vi "Query_Vizier.vi"(6 "Folder":path, 7 "wget":path, 8 "Width":dbl, 9 "Height":dbl, 10 "DEC":dbl, 11 "RA":dbl) -> (1 "error?":bool, 3 "Path2Image":path)   [LabVIEW 2019]
panel:
  out "standard output":string
  out "Final Name":string
  out "CMD Error":errorcluster
  out "standard error":string
  out "rm2 Error":errorcluster
  out "rm error":errorcluster
  out "Img Coords":cluster{"RA":dbl, "DEC":dbl}[](array[cluster]) {"DEC" format="%.2g"; "RA" format="%.2g"}
  out "complete command":string
  out "identifier":string
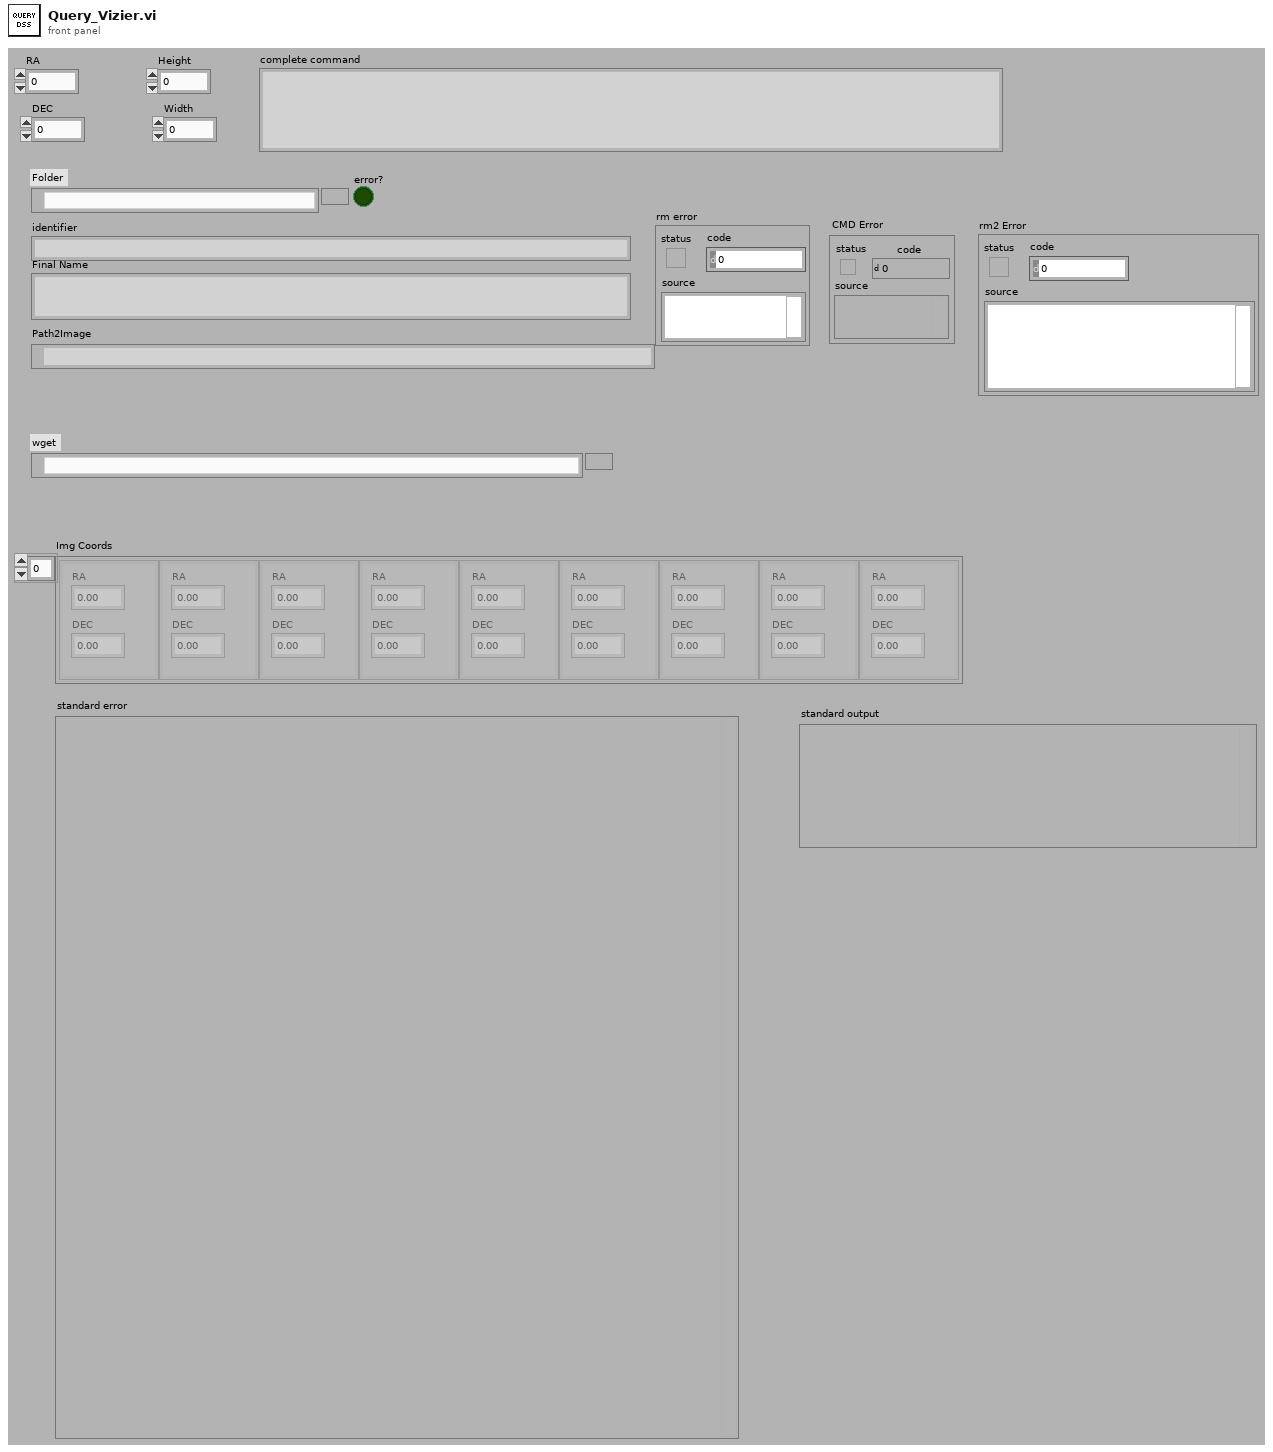
[diagram p1: front panel]
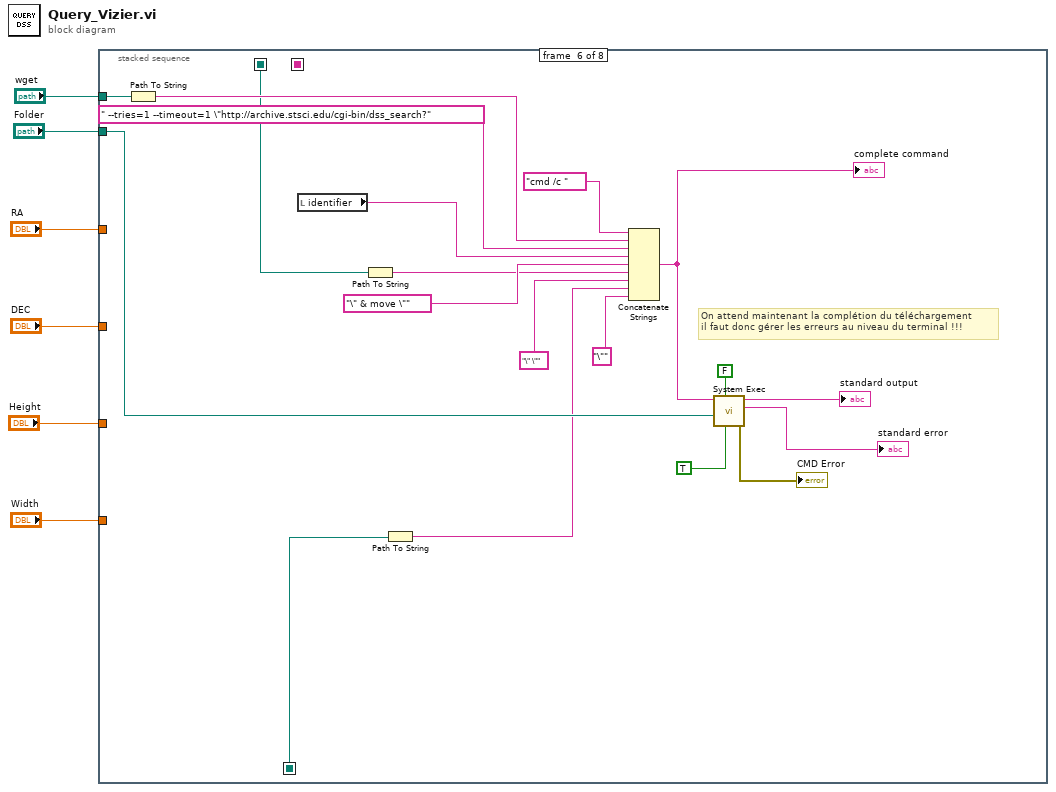
[diagram p0: block diagram]
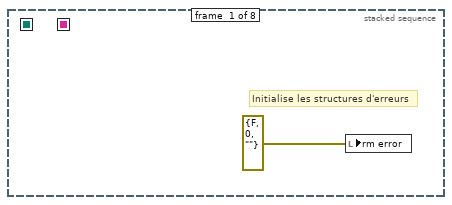
[diagram p2: hidden frame]
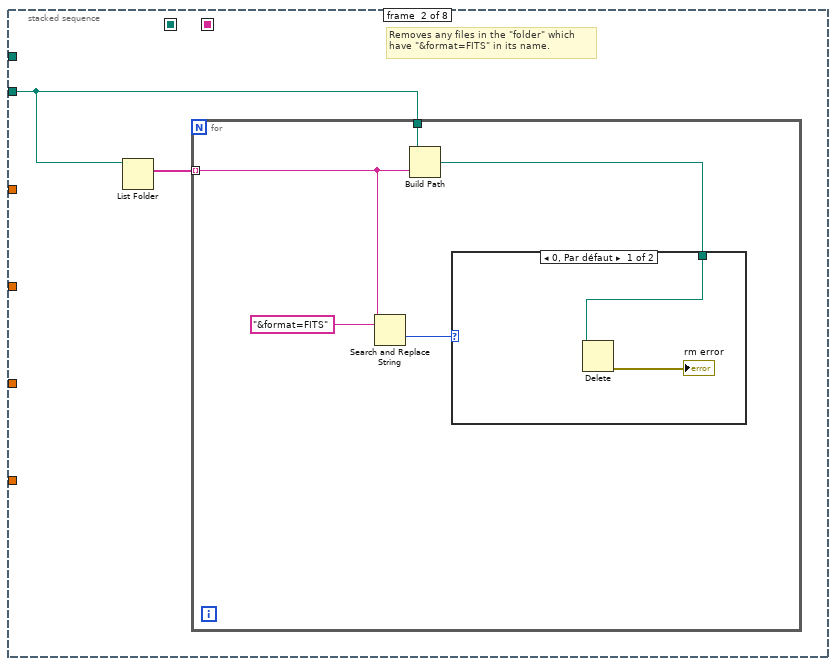
[diagram p3: hidden frame]
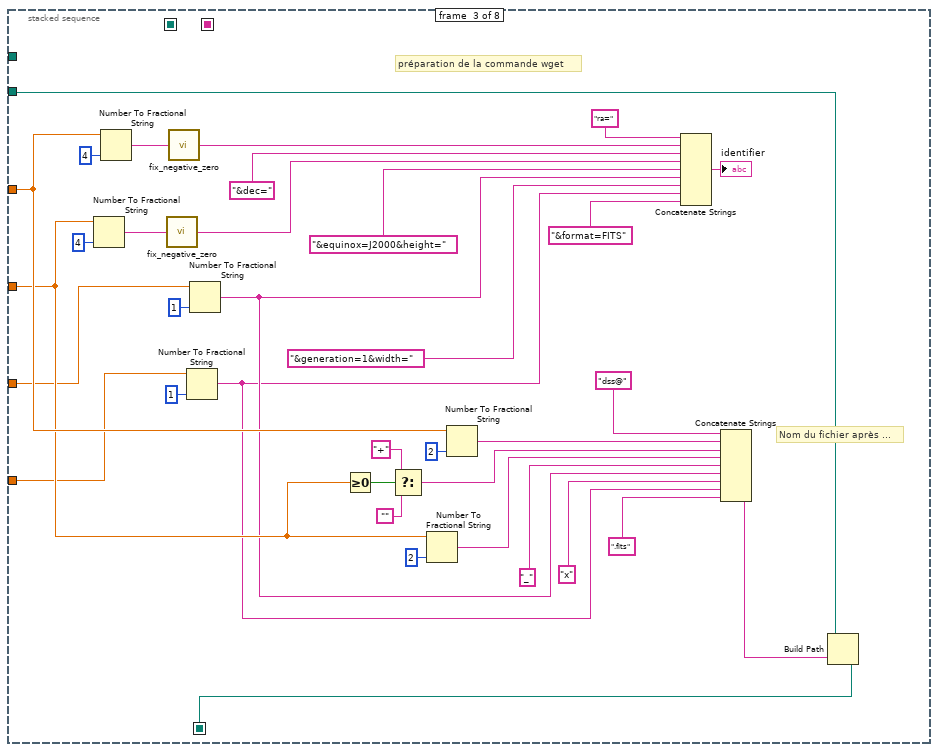
[diagram p5: hidden frame]
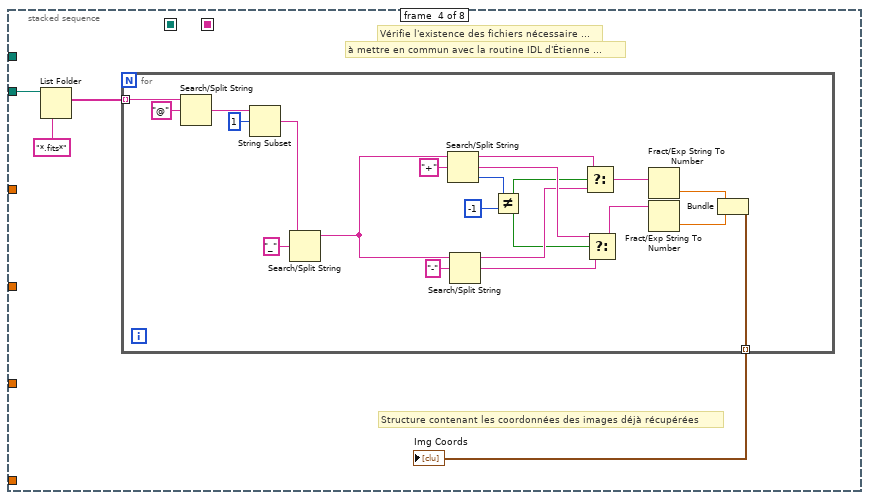
[diagram p6: hidden frame]
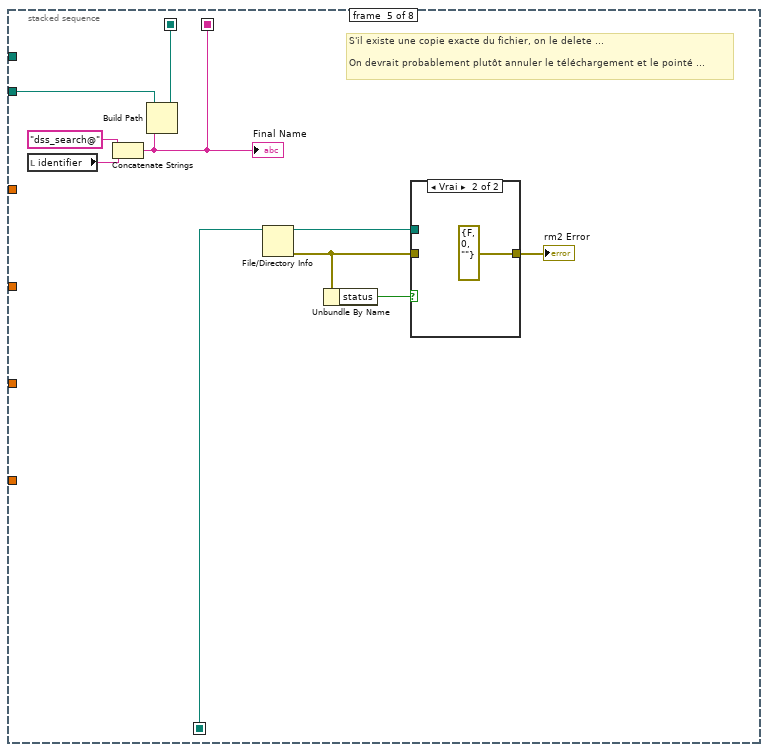
[diagram p7: hidden frame]
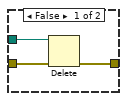
[diagram p8: hidden frame]
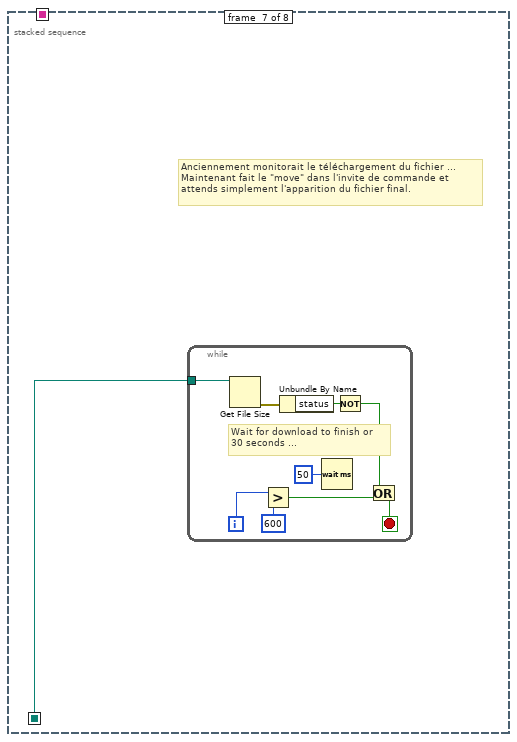
[diagram p9: hidden frame]
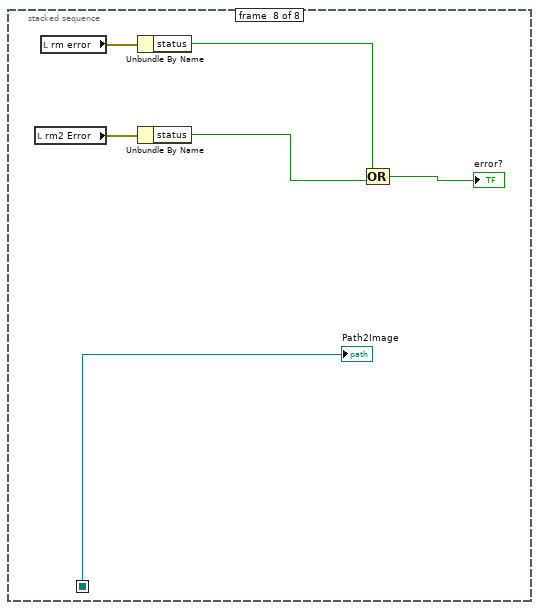
[diagram p10: hidden frame]
diagram:
  n1 = stacked-sequence {
    seq-local: [_ _ w20 _ _ _ _ _] -> [_ _ _ _ w77 w98 w110 w120]
    seq-local: [_ _ _ _ w82 _ _ _] -> [_ _ _ _ _ w97 _ _]
    seq-local: [_ _ _ _ w78 _ _ _] -> [_ _ _ _ _ _ _ _]
    tunnel: "Folder" -> [_ w8 w21 w55 w84 w109 _ _]
    tunnel: "RA" -> [_ _ w31 _ _ _ _ _]
    tunnel: "DEC" -> [_ _ w30 _ _ _ _ _]
    tunnel: "Height" -> [_ _ w29 _ _ _ _ _]
    tunnel: "Width" -> [_ _ w28 _ _ _ _ _]
    tunnel: "wget" -> [_ _ _ _ _ w104 _ _]
    frame #0 {
      # "Initialise les structures d'erreurs"
      n2 = local write "rm error"(errorcluster {"status"=FALSE, "code"=0, "source"=""} ("error out")) -> ()
    }
    frame #1 {
      # "Removes any files in the \"folder\" which\nhave \"&format=FITS\" in its name."
      n3 = List Folder(path=w8) -> (filenames=w9:string[])  [unwired: 3 in, 3 out]
      n4 = for {
        tunnel: w9 -> [w12] mode=indexing
        tunnel: w8 -> [w11]
        n5 = Search and Replace String(input string=w12, search string="&format=FITS") -> (offset past replacement=w13:i32)  [unwired: 6 in, 3 out]
        n6 = Build Path(base path=w11, name or relative path=w12) -> (appended path=w10:path)
        n7 = case shown="0, Par défaut" w13 {
          tunnel: w10 -> [w16 _]
          frame 0, Default {
            n8 = Delete(path (use dialog)=w16) -> (error out=→"rm error":errorcluster)  [unwired: 4 in, 2 out]
          }
          frame -1 {
          }
        }
      }
    }
    frame #2 {
      # "préparation de la commande wget"
      # "Nom du fichier après ..."
      n9 = Number To Fractional String(number=w30, precision (6)=i16 4) -> (F-format string=w33:string)  [unwired: 2 in]
      n10 = Number To Fractional String(number=w31, precision (6)=i16 4) -> (F-format string=w41:string)  [unwired: 2 in]
      n11 = call "fix_negative_zero.vi"("String IN"=w33) -> ("String OUT"=w17:string)
      n12 = call "fix_negative_zero.vi"("String IN"=w41) -> ("String OUT"=w18:string)
      n13 = Number To Fractional String(number=w28, precision (6)=i16 1) -> (F-format string=w23:string)  [unwired: 2 in]
      n14 = Number To Fractional String(number=w29, precision (6)=i16 1) -> (F-format string=w26:string)  [unwired: 2 in]
      n15 = Greater Or Equal To 0?(x=w30) -> (x >= 0?=w47:bool)
      n16 = Select(t="+" ("string"), s=w47, f="" ("string")) -> (s? t:f=w50:string)
      n17 = Number To Fractional String(number=w30, precision (6)=i16 2) -> (F-format string=w46:string)  [unwired: 2 in]
      n18 = Number To Fractional String(number=w31, precision (6)=i16 2) -> (F-format string=w45:string)  [unwired: 2 in]
      n19 = Concatenate Strings("ra=" ("string"), w18, "&dec=" ("string"), w17, "&equinox=J2000&height=" ("string"), w26, "&generation=1&width=" ("string"), w23, "&format=FITS" ("string")) -> (→"identifier":string)
      n20 = Concatenate Strings("dss@" ("string"), w45, w50, w46, "_" ("string"), w26, "x" ("string"), w23, ".fits" ("string")) -> (w22:string)
      n21 = Build Path(base path=w21, name or relative path=w22) -> (appended path=w20:path)
    }
    frame #3 {
      # "Structure contenant les coordonnées des images déjà récupérées"
      # "à mettre en commun avec la routine IDL d'Étienne ..."
      # "Vérifie l'existence des fichiers nécessaire ..."
      n22 = List Folder(path=w55, pattern="*.fits*") -> (filenames=w54:string[])  [unwired: 2 in, 3 out]
      n23 = for {
        tunnel: w54 -> [w76] mode=indexing
        tunnel: [w56] -> w52 mode=indexing
        n24 = Search/Split String(string=w76, search string/char (-)="@") -> (match + rest of string=w73:string)  [unwired: 1 in, 2 out]
        n25 = String Subset(string=w73, offset (0)=1) -> (substring=w71:string)  [unwired: 1 in]
        n26 = Search/Split String(string=w71, search string/char (-)="_") -> (substring before match=w66:string)  [unwired: 1 in, 2 out]
        n27 = Search/Split String(string=w66, search string/char (-)="+") -> (substring before match=w65:string, match + rest of string=w64:string, offset of match=w59:i32)  [unwired: 1 in]
        n28 = Search/Split String(string=w66, search string/char (-)="-") -> (substring before match=w62:string, match + rest of string=w63:string)  [unwired: 1 in, 1 out]
        n29 = Not Equal?(x=w59, y=-1) -> (x != y?=w57:bool)
        n30 = Select(t=w65, s=w57, f=w62) -> (s? t:f=w61:string)
        n31 = Select(t=w64, s=w57, f=w63) -> (s? t:f=w60:string)
        n32 = Fract/Exp String To Number(string=w61) -> (number=w69:dbl)  [unwired: 3 in, 1 out]
        n33 = Fract/Exp String To Number(string=w60) -> (number=w68:dbl)  [unwired: 3 in, 1 out]
        n34 = Bundle(w69, w68) -> (w56:cluster{dbl, dbl})  [unwired: 1 in]
      }
      "Img Coords" <- w52
    }
    frame #4 {
      # "S'il existe une copie exacte du fichier, on le delete ...\n\nOn devrait probablement plutôt annuler le téléchargement et le pointé ..."
      n35 = local read "identifier"() -> (w85:string)
      n36 = Concatenate Strings("dss_search@" ("string"), w85) -> (w78:string)
      "Final Name" <- w78
      n37 = Build Path(base path=w84, name or relative path=w78) -> (appended path=w82:path)
      n38 = File/Directory Info(path=w77) -> (path out=w81:path, error out=w79:errorcluster)  [unwired: 1 in, 5 out]
      n39 = Unbundle By Name(w79) -> ("status"=w80:bool)
      n40 = case shown="Vrai" w80 {
        tunnel: [w89 errorcluster {"status"=FALSE, "code"=0, "source"=""} ("error out")] -> w83
        tunnel: w81 -> [w88 _]
        tunnel: w79 -> [w87 _]
        frame False {
          n41 = Delete(path (use dialog)=w88, error in=w87) -> (error out=w89:errorcluster)  [unwired: 3 in, 2 out]
        }
        frame True {
        }
      }
      "rm2 Error" <- w83
    }
    frame #5 {
      # "On attend maintenant la complétion du téléchargement\nil faut donc gérer les erreurs au niveau du terminal !!!"
      n42 = Path To String(path=w104) -> (string=w103:string)
      n43 = local read "identifier"() -> (w99:string)
      n44 = Path To String(path=w97) -> (string=w96:string)
      n45 = Path To String(path=w98) -> (string=w94:string)
      n46 = Concatenate Strings("cmd /c " ("string"), w103, " --tries=1 --timeout=1 \"http://archive.stsci.edu/cgi-bin/dss_search?", w99, "\" & move \"" ("string"), w96, "\" \"" ("string"), w94, "\"" ("string")) -> (w106:string)
      "complete command" <- w106
      n47 = call <vilib>:"System Exec.vi"("run minimized? (F)"=TRUE, "wait until completion? (T)"=FALSE, "working directory"=w109, "command line"=w106) -> ("error out"=→"CMD Error":errorcluster, "standard error"=→"standard error":string, "standard output"=→"standard output":string)  [unwired: 4 in, 1 out]
    }
    frame #6 {
      # "Anciennement monitorait le téléchargement du fichier ...\nMaintenant fait le \"move\" dans l'invite de commande et \nattends simplement l'apparition du fichier final."
      n48 = while {
        tunnel: w110 -> [w119]
        i -> [w117]
        stop <- w115 stop-if-true
        # "Wait for download to finish or\n30 seconds ..."
        n49 = Get File Size(file=w119) -> (0:w111:errorcluster)  [unwired: 1 in, 2 out]
        n50 = Greater?(x=w117, y=600) -> (0:w114:bool)
        n51 = Unbundle By Name(w111) -> ("status"=w113:bool)
        n52 = Wait (ms)(milliseconds to wait=u32 50) -> ()  [unwired: 1 out]
        n53 = Not(x=w113) -> (.not. x?=w112:bool)
        n54 = Or(x=w112, y=w114) -> (x .or. y?=w115:bool)
      }
    }
    frame #7 {
      n55 = local read "rm2 Error"() -> (w124:errorcluster)
      n56 = local read "rm error"() -> (w125:errorcluster)
      n57 = Unbundle By Name(w125) -> ("status"=w123:bool)
      n58 = Unbundle By Name(w124) -> ("status"=w122:bool)
      n59 = Compound Arithmetic op=OR(w123, w122) -> (→"error?":bool)
      "Path2Image" <- w120
    }
  }
